vi "getDataFile.vi"(8 "error in (no error)":errorcluster, 10 "deviceType":T1, 11 "reference in":refnum<class "excelFile.lvclass">) -> (0 "error out":errorcluster, 3 "reference out":refnum<class "excelFile.lvclass">)   [LabVIEW 2016, in "excelFile.lvclass"]
uses:
  excelFile.lvclass
  SYS/Items Controller_llb/storageSheets.ctl
  SYS/Devices Controller_llb/deviceType.ctl
  <userlib>/Read_Excel_Values.llb/GetXL_CellValues_2D_String.vi
  SYS/Items Controller_llb/Items Controller.lvclass
  SYS/Devices Controller_llb/Devices Controller.lvclass
panel:
  out "data":string[][][](array[string])
  in  "storageSheets":T2
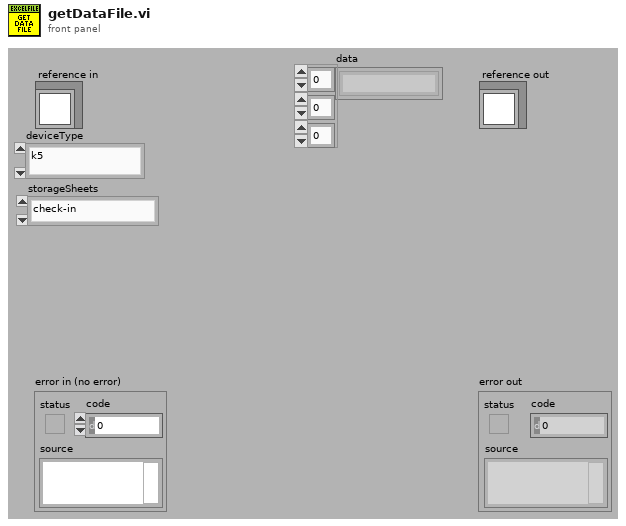
[diagram p1: front panel]
types:
  T1 = typedef "Devices Controller.lvclass/deviceType.ctl" = enum16{"k5", "k4b2", "fitmate", "cpet", "rmr", "bodyBoxPft", "bp", "pp"}
  T2 = typedef "Items Controller.lvclass/storageSheets.ctl" = enum16{"check-in", "check-out", "storage"}
  T3 = typedef "excelFile.lvclass/ObjectAttributesRef.ctl" = refnum<data-value>
  T4 = typedef "excelFile.lvclass/ObjectAttributes.ctl" = cluster{"MyAttribute":dbl, "path":string, "Refnum Excel":cluster{"Excel._Application":refnum<k7>, "Workbooks":refnum<k7>, "Open":refnum<k7>}, "data":string[][][], "save":bool, "fileType":T5, "rowsColor":u32[], "python_ref":refnum<class "python.lvclass">, "items_rows":i32[], "excel_range":i32[][], "TSR":cluster{"number":string, "TSR_path":path, "service_path":path, "email_to":string}, "excel_already_opened?":bool, "file_already_opened?":bool, "excel_protected_opened?":bool}
  T5 = typedef "excelFile.lvclass/fileType.ctl" = enum16{"devices", "items", "partsTracking", "TSR"}
  T6 = cluster{"Excel._Application":refnum<k7>, "Workbooks":refnum<k7>, "Open":refnum<k7>}
  T7 = cluster{"Excel._Application":refnum<k7>, "Workbooks":refnum<k7>, "Open":refnum<k7>, "Worksheets":refnum<k7>, "Excel._Worksheet":refnum<k7>}
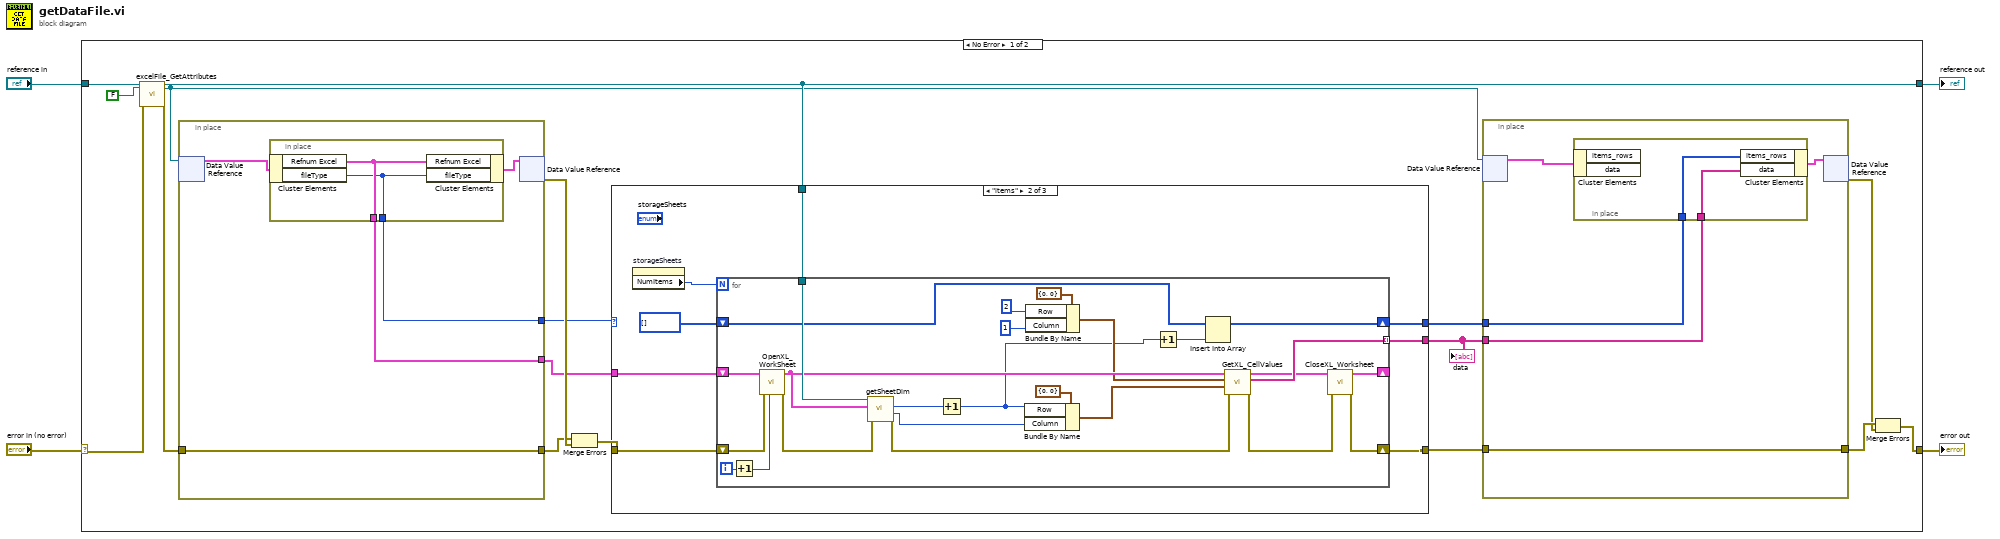
[diagram p0: block diagram]
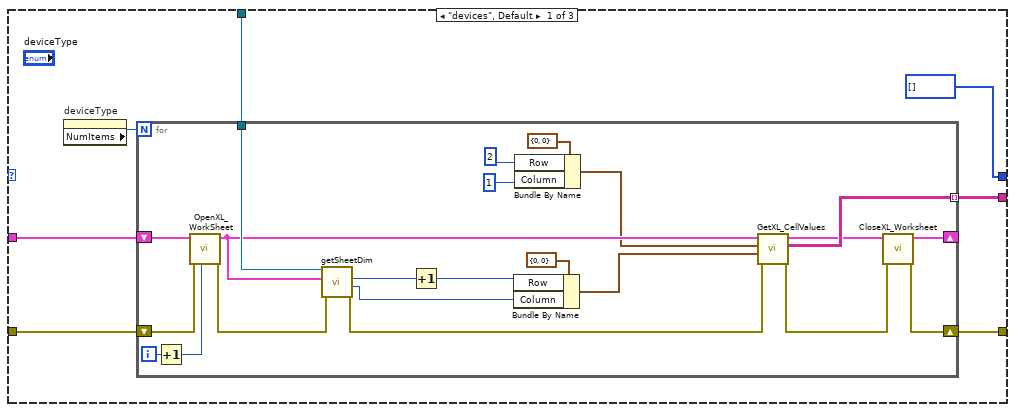
[diagram p2: hidden frame]
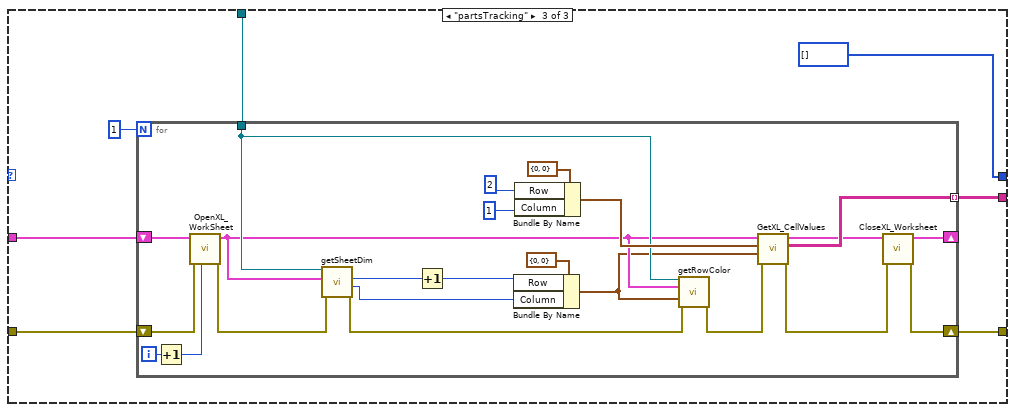
[diagram p3: hidden frame]
diagram:
  n1 = case shown="No Error" "error in (no error)" {
    selector: "error in (no error)" -> [w17 w129]
    tunnel: [w7 w129] -> w3
    tunnel: [w12 w128] -> w1
    tunnel: "reference in" -> [w19 w128]
    frame No Error {
      n2 = call "excelFile_GetAttributes.vi"("reference in"=w19, "return data? (T)"=FALSE, "error in (no error)"=w17) -> ("reference out"=w12:refnum<class "excelFile.lvclass">, "attributes ref"=w10:T3, "error out"=w16:errorcluster)  [unwired: 13 in, 1 out]
      n3 = in-place {
        in-place-border: w16 -> [w123]
        in-place-border: [w123] -> w20
        in-place-border: [w122] -> w13
        in-place-border: [w121] -> w14
        n4 = in-place-dvr #1(w10) -> (w124:T4)  [unwired: 1 out]
        n5 = in-place {
          in-place-border: [w127] -> w122
          in-place-border: [w126] -> w121
          n6 = in-place-cluster #2(w124) -> ("Refnum Excel"=w127:T6, "fileType"=w126:T5)
          n7 = in-place-cluster #2("Refnum Excel"=w127, "fileType"=w126) -> (w125:T4)
        }
        n8 = in-place-dvr #1(w125) -> (w21:errorcluster)  [unwired: 1 out]
      }
      n9 = Merge Errors(w20, w21) -> (w15:errorcluster)
      n10 = case shown="\"items\"" w14 {
        tunnel: w15 -> [w35 w65 w94]
        tunnel: [w34 w61 w93] -> w11
        tunnel: w13 -> [w33 w64 w95]
        tunnel: w12 -> [w32 w63 w97]
        tunnel: [w31 w62 w92] -> w5
        tunnel: [i32[] [] w58 i32[] []] -> w6
        frame "devices", Default {
          n11 = property on="deviceType" class="Enum (strict)"() -> ("NumItems"=w30:u32)  [unwired: 2 in, 2 out]
          n12 = for {
            N: w30 -> [_]
            shift-right: [w44] -> w34
            shift-left: w35 -> [w48]
            tunnel: w32 -> [w57]
            tunnel: [w38] -> w31 mode=indexing
            shift-right: [w45] -> _
            shift-left: w33 -> [w49]
            i -> [w50]
            n13 = Increment(x=w50) -> (x+1=w46:i32)
            n14 = call <userlib>:"OpenXL_WorkSheet.vi"("Sheet"=w46, "error in (no error)"=w48, "Refnum Cluster In"=w49) -> ("error out"=w47:errorcluster, "Refnum Cluster Out"=w43:T7)  [unwired: 7 in]
            n15 = call "getSheetDim.vi"("error in (no error)"=w47, "Refnum Cluster Out"=w43, "reference in"=w57) -> ("error out"=w40:errorcluster, "columnNumber"=w51:i32, "rowNumber"=w52:i32)  [unwired: 5 in, 1 out]
            n16 = Increment(x=w52) -> (x+1=w36:i32)
            n17 = Bundle By Name(cluster=cluster{"Column":i32, "Row":i32} {"Column"=0, "Row"=0} ("Start"), "Row"=w36, "Column"=w51) -> (w41:cluster{"Column":i32, "Row":i32})
            n18 = Bundle By Name(cluster=cluster{"Column":i32, "Row":i32} {"Column"=0, "Row"=0} ("Start"), "Row"=2 ("Column"), "Column"=1) -> (w42:cluster{"Column":i32, "Row":i32})
            n19 = call-poly <userlib>:"GetXL_CellValues.vi"("error in"=w40, "End"=w41, "Start"=w42, "Refnum Cluster In"=w43) -> ("error out"=w39:errorcluster, "data"=w38:string[][], "Refnum Cluster Out"=w37:T7)  [unwired: 5 in]
            n20 = call <userlib>:"CloseXL_Worksheet.vi"("error in (no error)"=w39, "Refnum Cluster In"=w37) -> ("error out"=w44:errorcluster, "Refnum Cluster Out"=w45:T6)  [unwired: 8 in]
          }
        }
        frame "items" {
          n21 = property on="storageSheets" class="Enum (strict)"() -> ("NumItems"=w60:u32)  [unwired: 2 in, 2 out]
          n22 = for {
            N: w60 -> [_]
            shift-right: [w77] -> w61
            shift-left: w65 -> [w81]
            tunnel: w63 -> [w90]
            tunnel: [w71] -> w62 mode=indexing
            shift-right: [w78] -> _
            shift-left: w64 -> [w82]
            shift-right: [w67] -> w58
            shift-left: i32[] [] -> [w66]
            i -> [w83]
            n23 = Increment(x=w83) -> (x+1=w79:i32)
            n24 = call <userlib>:"OpenXL_WorkSheet.vi"("Sheet"=w79, "error in (no error)"=w81, "Refnum Cluster In"=w82) -> ("error out"=w80:errorcluster, "Refnum Cluster Out"=w76:T7)  [unwired: 7 in]
            n25 = call "getSheetDim.vi"("error in (no error)"=w80, "Refnum Cluster Out"=w76, "reference in"=w90) -> ("error out"=w73:errorcluster, "columnNumber"=w84:i32, "rowNumber"=w85:i32)  [unwired: 5 in, 1 out]
            n26 = Increment(x=w85) -> (x+1=w69:i32)
            n27 = Bundle By Name(cluster=cluster{"Column":i32, "Row":i32} {"Column"=0, "Row"=0} ("Start"), "Row"=w69, "Column"=w84) -> (w74:cluster{"Column":i32, "Row":i32})
            n28 = Bundle By Name(cluster=cluster{"Column":i32, "Row":i32} {"Column"=0, "Row"=0} ("Start"), "Row"=2 ("Column"), "Column"=1) -> (w75:cluster{"Column":i32, "Row":i32})
            n29 = Increment(x=w69) -> (x+1=w68:i32)
            n30 = Insert Into Array(array=w66, new element=w68) -> (w67:i32[])  [unwired: 1 in]
            n31 = call-poly <userlib>:"GetXL_CellValues.vi"("error in"=w73, "End"=w74, "Start"=w75, "Refnum Cluster In"=w76) -> ("error out"=w72:errorcluster, "data"=w71:string[][], "Refnum Cluster Out"=w70:T7)  [unwired: 5 in]
            n32 = call <userlib>:"CloseXL_Worksheet.vi"("error in (no error)"=w72, "Refnum Cluster In"=w70) -> ("error out"=w77:errorcluster, "Refnum Cluster Out"=w78:T6)  [unwired: 8 in]
          }
        }
        frame "partsTracking" {
          n33 = for {
            N: 1 -> [_]
            shift-right: [w108] -> w93
            shift-left: w94 -> [w112]
            tunnel: w97 -> [w102]
            tunnel: [w105] -> w92 mode=indexing
            shift-right: [w109] -> _
            shift-left: w95 -> [w113]
            i -> [w114]
            n34 = Increment(x=w114) -> (x+1=w110:i32)
            n35 = call <userlib>:"OpenXL_WorkSheet.vi"("Sheet"=w110, "error in (no error)"=w112, "Refnum Cluster In"=w113) -> ("error out"=w111:errorcluster, "Refnum Cluster Out"=w101:T7)  [unwired: 7 in]
            n36 = call "getSheetDim.vi"("error in (no error)"=w111, "Refnum Cluster Out"=w101, "reference in"=w102) -> ("error out"=w99:errorcluster, "columnNumber"=w115:i32, "rowNumber"=w116:i32)  [unwired: 5 in, 1 out]
            n37 = Increment(x=w116) -> (x+1=w103:i32)
            n38 = Bundle By Name(cluster=cluster{"Column":i32, "Row":i32} {"Column"=0, "Row"=0} ("Start"), "Row"=w103, "Column"=w115) -> (w100:cluster{"Column":i32, "Row":i32})
            n39 = Bundle By Name(cluster=cluster{"Column":i32, "Row":i32} {"Column"=0, "Row"=0} ("Start"), "Row"=2 ("Column"), "Column"=1) -> (w107:cluster{"Column":i32, "Row":i32})
            n40 = call "getRowColor.vi"("reference in"=w102, "Refnum Cluster In"=w101, "End"=w100, "error in (no error)"=w99) -> ("error out"=w98:errorcluster)  [unwired: 10 in, 1 out]
            n41 = call-poly <userlib>:"GetXL_CellValues.vi"("error in"=w98, "End"=w100, "Start"=w107, "Refnum Cluster In"=w101) -> ("error out"=w106:errorcluster, "data"=w105:string[][], "Refnum Cluster Out"=w104:T7)  [unwired: 5 in]
            n42 = call <userlib>:"CloseXL_Worksheet.vi"("error in (no error)"=w106, "Refnum Cluster In"=w104) -> ("error out"=w108:errorcluster, "Refnum Cluster Out"=w109:T6)  [unwired: 8 in]
          }
        }
      }
      "data" <- w5
      n43 = in-place {
        in-place-border: w11 -> [w24]
        in-place-border: [w24] -> w9
        in-place-border: w5 -> [w23]
        in-place-border: w6 -> [w22]
        n44 = in-place-dvr #3(w10) -> (w25:T4)  [unwired: 1 out]
        n45 = in-place {
          in-place-border: w23 -> [w28]
          in-place-border: w22 -> [w27]
          n46 = in-place-cluster #4(w25) -> ()  [unwired: 2 out]
          n47 = in-place-cluster #4("items_rows"=w27, "data"=w28) -> (w26:T4)
        }
        n48 = in-place-dvr #3(w26) -> (w8:errorcluster)  [unwired: 1 out]
      }
      n49 = Merge Errors(w9, w8) -> (w7:errorcluster)
    }
    frame Error {
    }
  }
  "error out" <- w3
  "reference out" <- w1
